vi "Main.vi"(8 "error in (no error)":errorcluster, 11 "Example Class B in":refnum<class "ExampleClassB.lvclass">) -> (0 "error out":errorcluster, 3 "Example Class B out":refnum<class "ExampleClassB.lvclass">)   [LabVIEW 2012, in "ExampleClassB.lvclass"]
doc: "Main VI and GUI of this component."
uses:
  ExampleClassB.lvclass
  <vilib>/Distrio/Murmex/InitialiseMessage/InitialiseMessage.lvclass
  ExampleClassB.lvclass/ExampleClassB.ctl
  <vilib>/Distrio/Murmex/ConfigureMessage/ConfigureMessage.lvclass
  <vilib>/Distrio/Murmex/TerminateMessage/TerminateMessage.lvclass
  <vilib>/Distrio/Murmex/Murmex/Set configure at initialise.vi
  <vilib>/Distrio/Murmex/Murmex/Set VI reference.vi
  <vilib>/Distrio/Murmex/Murmex/Get ID.vi
  <vilib>/Distrio/Murmex/Murmex/Set log reference.vi
  <vilib>/Distrio/Murmex/Murmex/Murmex.lvclass
panel:
  out "Log":string
  in  "Tab Control":enum32{"User", "Debug"}(tab)
  in  "button:configure":bool
  out "Received data":dbl[][](graph)
  in  "button:quit":bool
  out "Expected number of samples":i32
  in  "component ID":string
  out "terminated?":bool
  out "main loop counter":i32
  out "component B":refnum<class "ExampleClassB.lvclass">
  # "IMPORTANT: When starting this VI directly, enter its ID on the Debug tab."
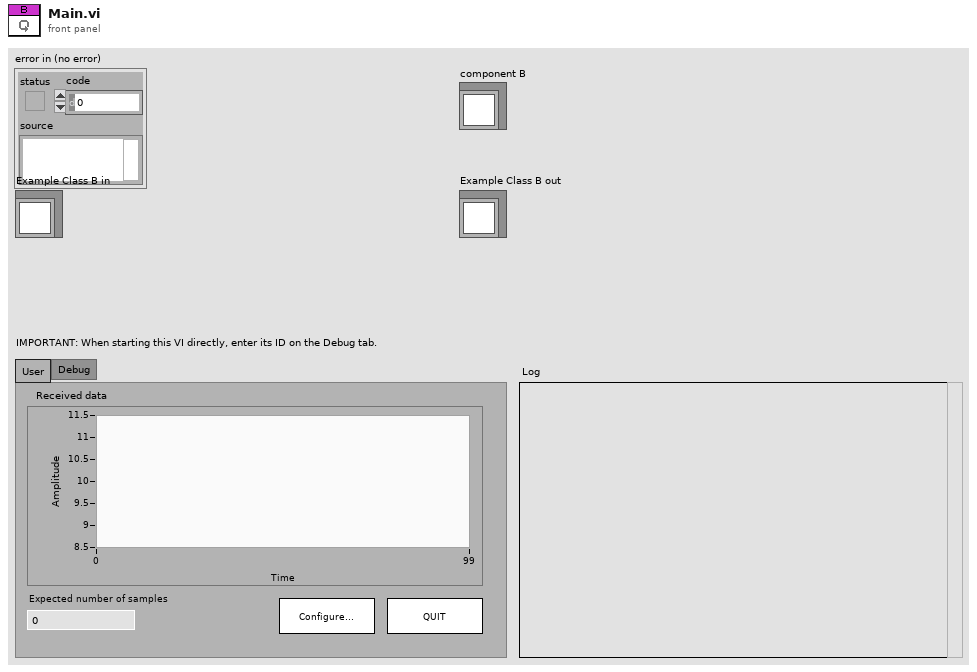
[diagram p1: front panel]
types:
  T1 = enum8{"Enabled", "Disabled", "Disabled and Grayed Out"}
  T2 = typedef "Murmex.lvclass/command_enum.ctl" = enum16{"null", "initialise", "reset", "terminate", "acknowledge", "update", "inspect", "inform", "proceed", "start", "stop", "fetch", "configure", "generic"}
  T3 = typedef "Murmex.lvclass/Event type enumerations.ctl" = enum16{"before", "after"}
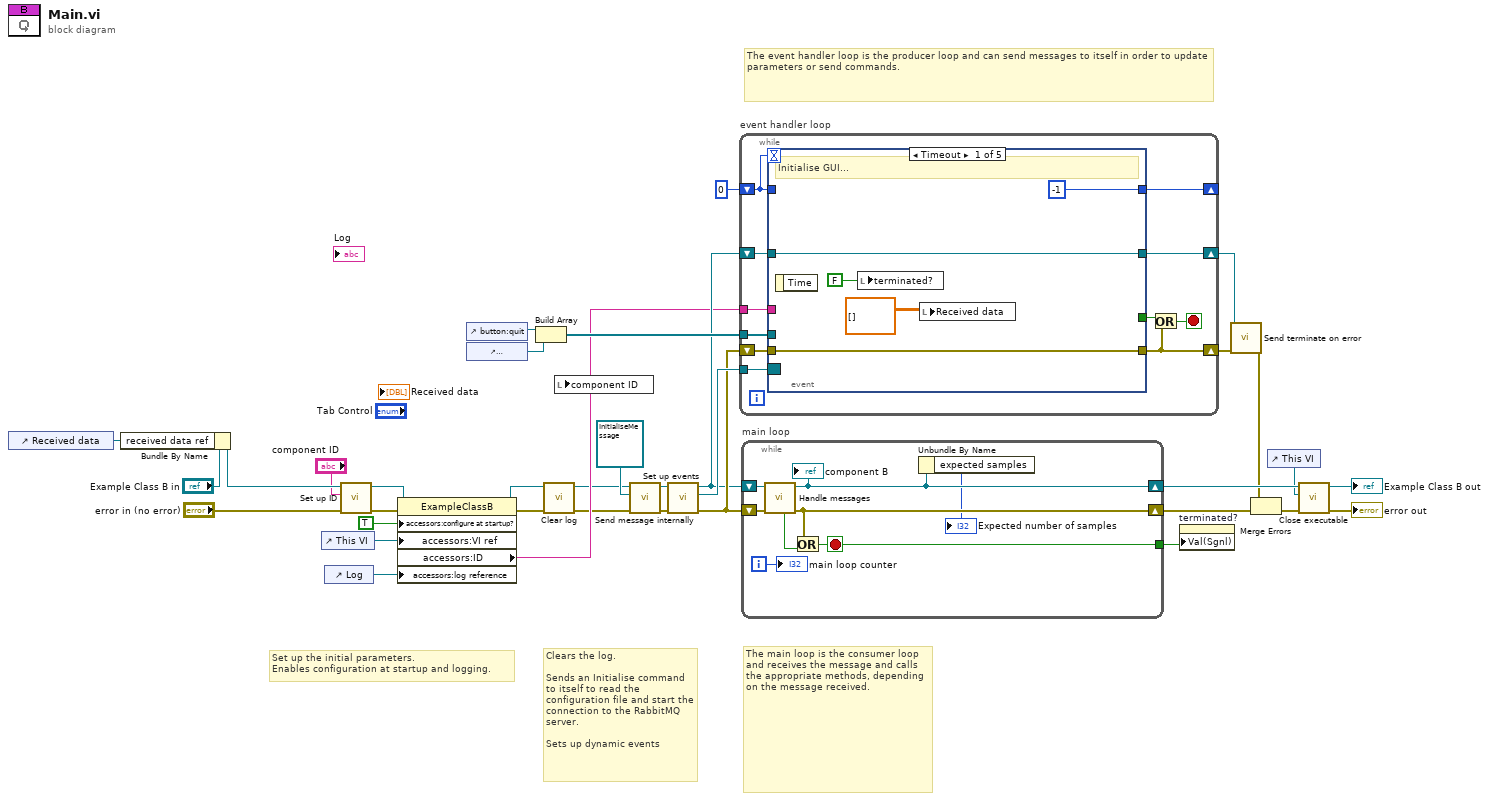
[diagram p0: block diagram]
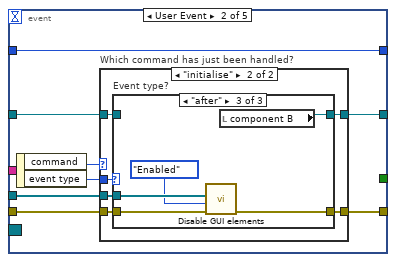
[diagram p2: hidden frame]
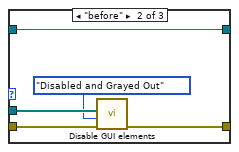
[diagram p5: hidden frame]
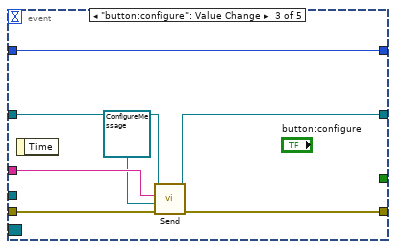
[diagram p6: hidden frame]
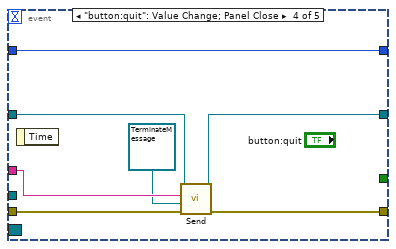
[diagram p7: hidden frame]
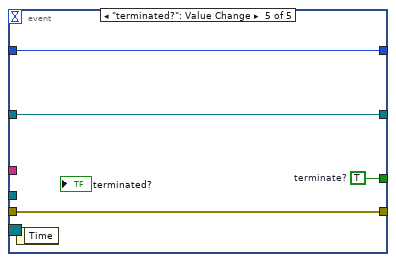
[diagram p8: hidden frame]
diagram:
  # "The event handler loop is the producer loop and can send messages to itself in order to update parameters or send commands."
  # "The main loop is the consumer loop and receives the message and calls the appropriate methods, depending on the message received."
  # "Clears the log.\n\nSends an Initialise command to itself to read the configuration file and start the connection to the RabbitMQ server.\n\nSets up dynamic events"
  # "Set up the initial parameters. \nEnables configuration at startup and logging."
  n1 = control-ref of="Received data"() -> (w31:refnum<vi>)
  n2 = Bundle By Name(cluster="Example Class B in", "received data ref"=w31) -> (w32:refnum<class "ExampleClassB.lvclass">)
  n3 = control-ref of="This VI"() -> (w9:refnum<vi>)
  n4 = control-ref of="Log"() -> (w5:refnum<vi>)
  n5 = call <vilib>:"Set up ID.vi"("error in (no error)"="error in (no error)", "component ID"="component ID", "MurmexBase in"=w32) -> ("error out"=w8:errorcluster, "MurmexBase out"=w7:refnum<class "ExampleClassB.lvclass">)  [unwired: 6 in, 1 out]
  n6 = property class="ExampleClassB"(reference=w7, error in=w8, "accessors:configure at startup?"=TRUE ("configure at startup?"), "accessors:VI ref"=w9, "accessors:log reference"=w5) -> (reference out=w4:refnum<class "ExampleClassB.lvclass">, error out=w2:errorcluster, "accessors:ID"=w6:string)
  n7 = control-ref of="button:quit"() -> (w19:refnum<vi>)
  n8 = control-ref of="button:configure"() -> (w18:refnum<vi>)
  n9 = Build Array(w19, w18) -> (w20:refnum<vi>[])
  n10 = call <vilib>:"Clear log.vi"("error in (no error)"=w2, "MurmexBase in"=w4) -> ("error out"=w1:errorcluster, "MurmexBase out"=w3:refnum<class "ExampleClassB.lvclass">)  [unwired: 8 in]
  n11 = local write "component ID"(w6) -> ()
  n12 = call <vilib>:"Send message internally.vi"("error in (no error)"=w1, "Message"=refnum<class "InitialiseMessage.lvclass"> refnum ("InitialiseMessage.lvclass"), "Murmex in"=w3) -> ("error out"=w23:errorcluster, "Murmex out"=w21:refnum<class "ExampleClassB.lvclass">)  [unwired: 7 in]
  n13 = call <vilib>:"Set up events.vi"("error in (no error)"=w23, "MurmexBase in"=w21) -> ("error out"=w22:errorcluster, "Event Registration Refnum"=w24:refnum<event-registration>, "MurmexBase out"=w10:refnum<class "ExampleClassB.lvclass">)  [unwired: 7 in]
  n14 = while "event handler loop" {
    shift-right: [w44] -> _
    shift-left: 0 -> [w45]
    shift-right: [w36] -> w14
    shift-left: w22 -> [w46]
    tunnel: w24 -> [w43]
    tunnel: w20 -> [w42]
    tunnel: w6 -> [w41]
    shift-right: [w40] -> w11
    shift-left: w10 -> [w39]
    stop <- w37 stop-if-true
    n15 = event shown="[0] Timeout" {
      selector: w43 -> [_ _ _ _ _]
      dyn-events: _ -> [_ _ _ _ _]
      timeout: w45 -> [_ _ _ _ _]
      tunnel: [_ _ _ _ w95] -> w38
      tunnel: [w48 w56 w82 w89 w97] -> w36
      tunnel: w46 -> [w48 w57 w83 w90 w97]
      tunnel: [-1 w59 w86 w93 w96] -> w44
      tunnel: w45 -> [_ w59 w86 w93 w96]
      tunnel: w42 -> [_ w55 _ _ _]
      tunnel: w41 -> [_ _ w85 w92 _]
      tunnel: [w47 w53 w80 w87 w94] -> w40
      tunnel: w39 -> [w47 w52 w81 w88 w94]
      event Timeout {
        # "Initialise GUI..."
        n16 = event-data() -> ()  [unwired: 1 in, 1 out]
        n17 = local write "terminated?"(FALSE ("terminated?")) -> ()
        n18 = local write "Received data"(dbl[][] [] ("Received data")) -> ()
      }
      event User Event {
        n19 = event-data() -> ("command"=w58:T2, "event type"=w54:T3)  [unwired: 1 in]
        n20 = case "Which command has just been handled?" shown="\"initialise\"" w58 {
          tunnel: w57 -> [w61 w66]
          tunnel: [w61 w64] -> w56
          tunnel: w55 -> [_ w65]
          tunnel: w54 -> [_ w67]
          tunnel: [w60 w63] -> w53
          tunnel: w52 -> [w60 w62]
          frame Default {
          }
          frame "initialise" {
            n21 = case "Event type?" shown="\"after\"" w67 {
              tunnel: w66 -> [w69 w74 w76]
              tunnel: w65 -> [_ w72 w79]
              tunnel: [w69 w73 w77] -> w64
              tunnel: [w68 w70 w75] -> w63
              tunnel: w62 -> [w68 w70 _]
              frame Default {
              }
              frame "before" {
                n22 = call <vilib>:"Disable GUI elements.vi"("error in (no error)"=w74, "enabled state"=T1."Disabled and Grayed Out" ("Disabled"), "control refs"=w72) -> ("error out"=w73:errorcluster)  [unwired: 8 in]
              }
              frame "after" {
                n23 = call <vilib>:"Disable GUI elements.vi"("error in (no error)"=w76, "enabled state"=T1."Enabled" ("Disabled"), "control refs"=w79) -> ("error out"=w77:errorcluster)  [unwired: 8 in]
                n24 = local read "component B"() -> (w75:refnum<class "ExampleClassB.lvclass">)
              }
            }
          }
        }
      }
      event "button:configure": Value Change {
        n25 = event-data() -> ()  [unwired: 1 in, 1 out]
        n26 = call <vilib>:"Send.vi"("error in (no error)"=w83, "Message"=refnum<class "ConfigureMessage.lvclass"> refnum ("ConfigureMessage.lvclass"), "recipient"=w85, "Murmex in"=w81) -> ("error out"=w82:errorcluster, "Murmex out"=w80:refnum<class "ExampleClassB.lvclass">)  [unwired: 6 in]
      }
      event "button:quit": Value Change; Panel Close {
        n27 = event-data() -> ()  [unwired: 1 in, 1 out]
        n28 = call <vilib>:"Send.vi"("error in (no error)"=w90, "Message"=refnum<class "TerminateMessage.lvclass"> refnum ("TerminateMessage.lvclass"), "recipient"=w92, "Murmex in"=w88) -> ("error out"=w89:errorcluster, "Murmex out"=w87:refnum<class "ExampleClassB.lvclass">)  [unwired: 6 in]
      }
      event "terminated?": Value Change {
        w95 = TRUE  # terminate?
        n29 = event-data() -> ()  [unwired: 1 in, 1 out]
      }
    }
    n30 = Or(x=w38, y=w36) -> (x .or. y?=w37:bool)
  }
  n31 = while "main loop" {
    tunnel: [w101] -> w25
    shift-right: [w102] -> w29
    shift-left: w22 -> [w105]
    shift-right: [w99] -> w16
    shift-left: w10 -> [w104]
    i -> [w100]
    stop <- w101 stop-if-true
    n32 = call <vilib>:"Handle messages.vi"("error in (no error)"=w105, "Murmex in"=w104) -> ("error out"=w102:errorcluster, "Murmex out"=w99:refnum<class "ExampleClassB.lvclass">, "terminated?"=w103:bool)  [unwired: 7 in]
    "component B" <- w99
    n33 = Or(x=w102, y=w103) -> (x .or. y?=w101:bool)
    n34 = Unbundle By Name(w99) -> ("expected samples"=→"Expected number of samples":i32)
    "main loop counter" <- w100
  }
  n35 = property on="terminated?" class="Bool (strict)"("Val(Sgnl)"=w25) -> ()  [unwired: 2 in, 2 out]
  n36 = call <vilib>:"Send terminate on error.vi"("error in (no error)"=w14, "Murmex in"=w11) -> ("error out"=w13:errorcluster)  [unwired: 8 in, 1 out]
  n37 = Merge Errors(w13, w29) -> (w17:errorcluster)
  n38 = control-ref of="This VI"() -> (w15:refnum<vi>)
  n39 = call <vilib>:"Close executable.vi"("error in (no error)"=w17, "main VI ref (optional)"=w15, "MurmexBase in"=w16) -> ("error out"=→"error out":errorcluster, "MurmexBase out"=→"Example Class B out":refnum<class "ExampleClassB.lvclass">)  [unwired: 7 in]
